vi "PixyCam_GetStart.vi"(4 "error in":errorcluster, 7 "PixyCamDevRef":T1) -> (0 "error out":errorcluster, 2 "WordType":u16(ring)=43605 items=["PIXY_START_WORD"=43605, "PIXY_START_WORD_CC"=43606, "PIXY_START_WORDX"=21930], 3 "PixyCamDevRef Out":T1)   [LabVIEW 2016, in "PixyCam_LabVIEW.lvlib"]
uses:
  PixyCam_LabVIEW.lvlib
  PixyCam_DevRef.ctl
  PixyCam_SPI_DevRef.ctl
  <vilib>/Rock Robotics/WPI/SPI/WPI_SPIDevRef.ctl
  <vilib>/Rock Robotics/SystemInterfaces/spilib/spi_bus.ctl
  PixyCam_CommMode.ctl
  <vilib>/Utility/SystemLogging/NI_SystemLogging.lvlib
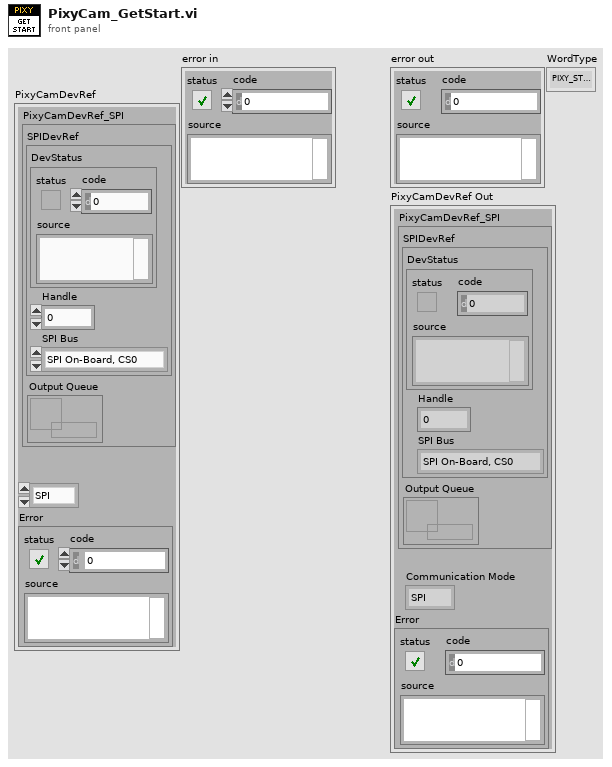
[diagram p1: front panel]
types:
  T1 = typedef "PixyCam_LabVIEW.lvlib/PixyCam_DevRef.ctl" = cluster{"PixyCamDevRef_SPI":T2, "Communication Mode":T5, "Error":errorcluster}
  T2 = typedef "PixyCam_LabVIEW.lvlib/PixyCam_SPI_DevRef.ctl" = cluster{"SPIDevRef":T3, "Output Queue":refnum<queue>}
  T3 = typedef "WPI_SPIDevRef.ctl" = cluster{"DevStatus":errorcluster, "Handle":i32, "SPI Bus":T4}
  T4 = typedef "spi_bus.ctl" = enum16{"SPI On-Board, CS0", "SPI On-Board, CS1", "SPI On-Board, CS2", "SPI On-Board, CS3", "SPI MXP", "Invalid"}
  T5 = typedef "PixyCam_LabVIEW.lvlib/PixyCam_CommMode.ctl" = enum16{"SPI", "I2C", "UART", "Analog", "Digital"}
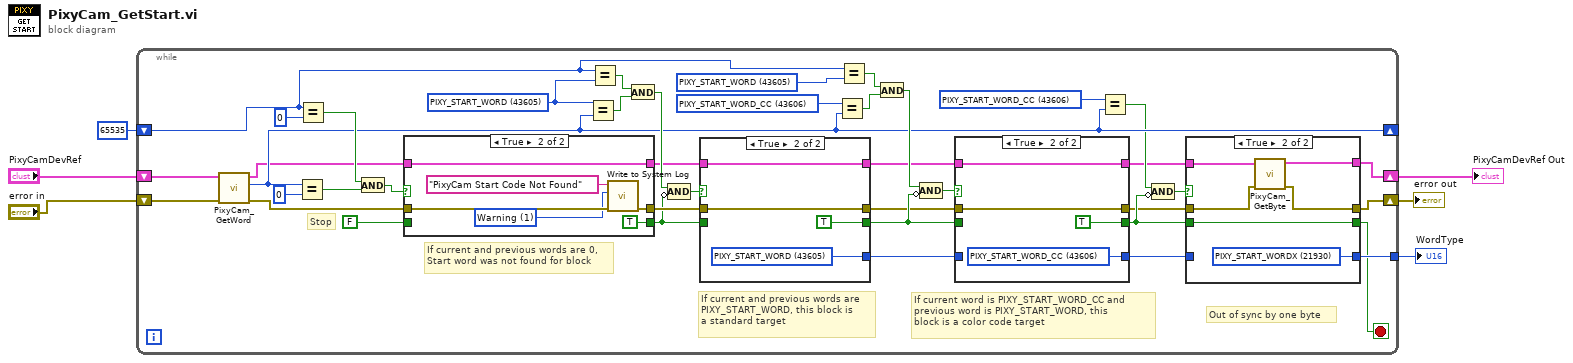
[diagram p0: block diagram]
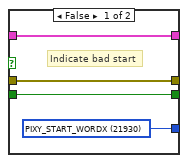
[diagram p4: hidden frame]
diagram:
  n1 = while {
    shift-right: [w8] -> w3
    shift-left: "PixyCamDevRef" -> [w47]
    shift-right: [w13] -> w4
    shift-left: "error in" -> [w46]
    shift-right: [w21] -> _
    shift-left: u16 65535 ("Word Out") -> [w29]
    tunnel: [w16] -> w1
    stop <- w7 stop-if-true
    w22 = u16 43606 items=["PIXY_START_WORD"=43605, "PIXY_START_WORD_CC"=43606, "PIXY_START_WORDX"=21930] ("IDWord")
    w28 = u16 43605 items=["PIXY_START_WORD"=43605, "PIXY_START_WORD_CC"=43606, "PIXY_START_WORDX"=21930] ("IDWord")
    w30 = u16 43606 items=["PIXY_START_WORD"=43605, "PIXY_START_WORD_CC"=43606, "PIXY_START_WORDX"=21930] ("IDWord")
    w40 = u16 43605 items=["PIXY_START_WORD"=43605, "PIXY_START_WORD_CC"=43606, "PIXY_START_WORDX"=21930] ("IDWord")
    # "Out of sync by one byte"
    # "If current word is PIXY_START_WORD_CC and\nprevious word is PIXY_START_WORD, this\nblock is a color code target"
    # "If current and previous words are\nPIXY_START_WORD, this block is\na standard target"
    # "Stop"
    # "If current and previous words are 0,\nStart word was not found for block"
    n2 = call "PixyCam_GetWord.vi"("error in"=w46, "PixyCamDevRef"=w47) -> ("error out"=w41:errorcluster, "Word Out"=w21:u16, "PixyCamDevRefOut"=w12:T1)  [unwired: 3 in]
    n3 = Equal?(x=w21, y=u16 0) -> (x = y?=w42:bool)
    n4 = Equal?(x=w29, y=u16 0) -> (x = y?=w43:bool)
    n5 = And(x=w43, y=w42) -> (x .and. y?=w36:bool)
    n6 = case shown="True" w36 {
      tunnel: w41 -> [w76 w82]
      tunnel: [w76 w80] -> w34
      tunnel: FALSE -> [w75 _]
      tunnel: [w75 TRUE] -> w32
      tunnel: w12 -> [w74 w78]
      tunnel: [w74 w78] -> w11
      frame False {
      }
      frame True {
        w77 = 1 items=["Error", "Warning", "Informational"] ("severity")
        n7 = call <vilib>:"Write to System Log.vi"("error in (no error)"=w82, "severity"=w77, "message"="PixyCam Start Code Not Found") -> ("error out"=w80:errorcluster)  [unwired: 8 in]
      }
    }
    n8 = Equal?(x=w40, y=w21) -> (x = y?=w38:bool)
    n9 = Equal?(x=w29, y=w40) -> (x = y?=w39:bool)
    n10 = And(x=w39, y=w38) -> (x .and. y?=w37:bool)
    n11 = Compound Arithmetic op=AND(w37, invert w32) -> (w35:bool)
    n12 = case shown="True" w35 {
      tunnel: w34 -> [w67 w71]
      tunnel: w32 -> [w69 _]
      tunnel: [w69 TRUE] -> w24
      tunnel: [w68 w73] -> w23
      tunnel: [w67 w71] -> w15
      tunnel: w11 -> [w66 w70]
      tunnel: [w66 w70] -> w10
      frame False {
        w68 = u16 21930 items=["PIXY_START_WORD"=43605, "PIXY_START_WORD_CC"=43606, "PIXY_START_WORDX"=21930] ("WordType 2")
        # "Indicate bad start"
      }
      frame True {
        w73 = u16 43605 items=["PIXY_START_WORD"=43605, "PIXY_START_WORD_CC"=43606, "PIXY_START_WORDX"=21930] ("WordType 2")
      }
    }
    n13 = Equal?(x=w30, y=w21) -> (x = y?=w31:bool)
    n14 = Equal?(x=w29, y=w28) -> (x = y?=w27:bool)
    n15 = And(x=w27, y=w31) -> (x .and. y?=w26:bool)
    n16 = Compound Arithmetic op=AND(w26, invert w24) -> (w25:bool)
    n17 = case shown="True" w25 {
      tunnel: w24 -> [w61 _]
      tunnel: [w61 TRUE] -> w18
      tunnel: [w60 w65] -> w17
      tunnel: w23 -> [w60 _]
      tunnel: w15 -> [w59 w63]
      tunnel: [w59 w63] -> w14
      tunnel: w10 -> [w58 w62]
      tunnel: [w58 w62] -> w9
      frame False {
      }
      frame True {
        w65 = u16 43606 items=["PIXY_START_WORD"=43605, "PIXY_START_WORD_CC"=43606, "PIXY_START_WORDX"=21930] ("WordType 2")
      }
    }
    n18 = Equal?(x=w22, y=w21) -> (x = y?=w20:bool)
    n19 = Compound Arithmetic op=AND(w20, invert w18) -> (w19:bool)
    n20 = case shown="True" w19 {
      tunnel: w18 -> [w51 w56]
      tunnel: [w51 w56] -> w7
      tunnel: [w50 w57] -> w16
      tunnel: w17 -> [w50 _]
      tunnel: w14 -> [w49 w53]
      tunnel: [w49 w52] -> w13
      tunnel: w9 -> [w48 w55]
      tunnel: [w48 w54] -> w8
      frame False {
      }
      frame True {
        w57 = u16 21930 items=["PIXY_START_WORD"=43605, "PIXY_START_WORD_CC"=43606, "PIXY_START_WORDX"=21930] ("WordType 2")
        n21 = call "PixyCam_GetByte.vi"("error in"=w53, "PixyCamDevRef"=w55) -> ("error out"=w52:errorcluster, "PixyCamDevRefOut"=w54:T1)  [unwired: 3 in, 1 out]
      }
    }
  }
  "error out" <- w4
  "PixyCamDevRef Out" <- w3
  "WordType" <- w1
